vi "Power On.vi"(8 "error in (no error)":errorcluster, 11 "Dual Fan in":refnum<class "Dual Fan.lvclass">) -> (0 "error out":errorcluster, 3 "Dual Fan out":refnum<class "Dual Fan.lvclass">)   [LabVIEW 2012, in "Dual Fan.lvlib" / "Dual Fan.lvclass"]
uses:
  Dual Fan.lvclass
  Dual Fan.lvclass/Dual Fan.ctl
  Simulation/Simulation Data_Global.vi
  Simulation/Simulation.lvlib
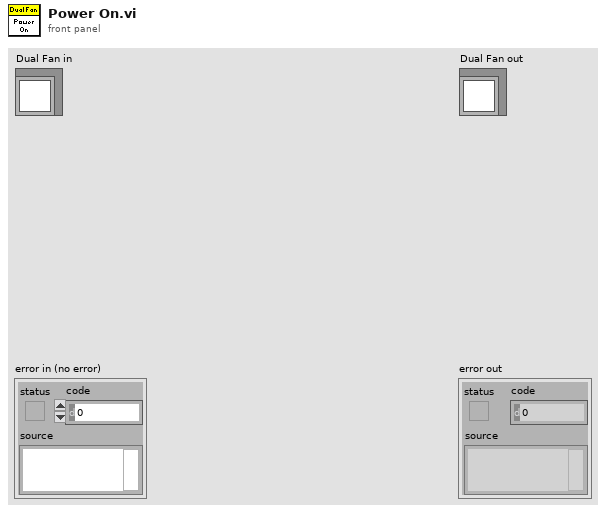
[diagram p1: front panel]
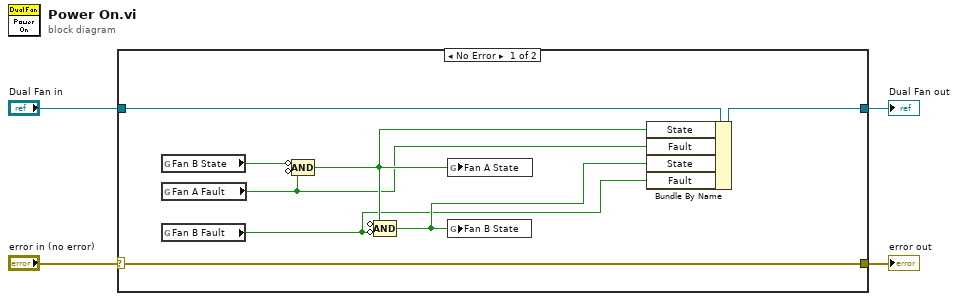
[diagram p0: block diagram]
diagram:
  n1 = case shown="No Error" "error in (no error)" {
    selector: "error in (no error)" -> [w12 w14]
    tunnel: [w12 w14] -> w3
    tunnel: [w10 w13] -> w1
    tunnel: "Dual Fan in" -> [w11 w13]
    frame No Error {
      n2 = global read "Simulation Data_Global.vi" "Fan B State"() -> (w5:bool)
      n3 = global read "Simulation Data_Global.vi" "Fan A Fault"() -> (w7:bool)
      n4 = global read "Simulation Data_Global.vi" "Fan B Fault"() -> (w6:bool)
      n5 = Compound Arithmetic op=AND(invert w5, invert w7) -> (w8:bool)
      n6 = Compound Arithmetic op=AND(invert w8, invert w6) -> (w9:bool)
      n7 = global write "Simulation Data_Global.vi" "Fan A State"(w8) -> ()
      n8 = global write "Simulation Data_Global.vi" "Fan B State"(w9) -> ()
      n9 = Bundle By Name(cluster=w11, "State"=w8, "Fault"=w7, "State"=w9, "Fault"=w6) -> (w10:refnum<class "Dual Fan.lvclass">)
    }
    frame Error {
    }
  }
  "error out" <- w3
  "Dual Fan out" <- w1
